vi "Get Column Widths.vi"(8 "error in (no error)":errorcluster, 10 "NewBnds":T1, 11 "Multicolumn List Box View Model In":refnum<class "Process Tree View Model.lvclass">) -> (0 "error out":errorcluster, 2 "Widths":i32[](array[numeric]), 3 "Multicolumn List Box View Model Out":refnum<class "Process Tree View Model.lvclass">)   [LabVIEW 2020, in "Process Tree View Model.lvclass"]
uses:
  Process Tree View Model.lvclass
  <vilib>/Utility/miscctls.llb/LVRectTypeDef.ctl
  Process Tree View Model.lvclass/Process Tree View Model.ctl
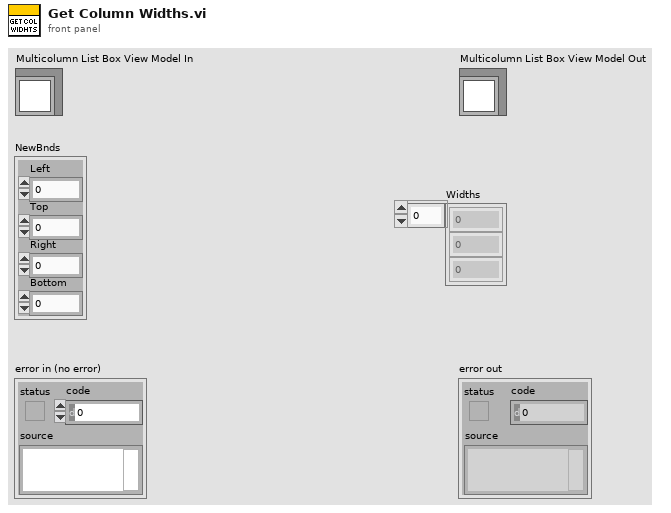
[diagram p1: front panel]
types:
  T1 = typedef "LVRectTypeDef.ctl" = cluster{"Left":i16, "Top":i16, "Right":i16, "Bottom":i16}
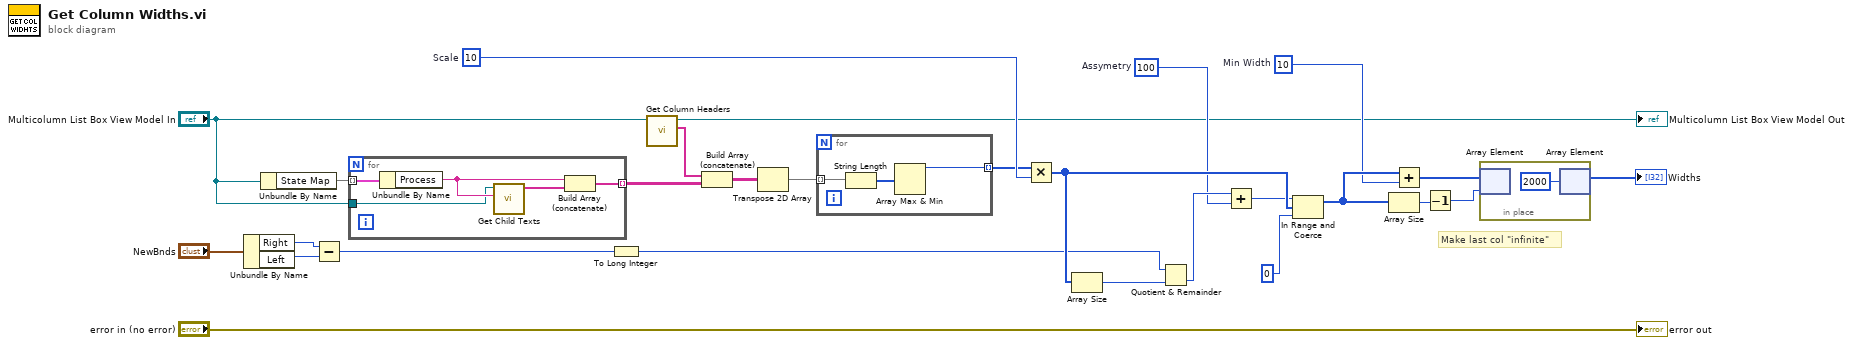
[diagram p0: block diagram]
diagram:
  w9 = 100  # Assymetry
  w11 = 10  # Min Width
  w26 = 10  # Scale
  # "Make last col \"infinite\""
  n1 = Unbundle By Name("NewBnds") -> ("Right"=w20:i16, "Left"=w19:i16)
  n2 = Unbundle By Name("Multicolumn List Box View Model In") -> ("State Map"=w1:map{string, string})
  n3 = Subtract(x=w20, y=w19) -> (x-y=w18:i16)
  n4 = for {
    tunnel: w1 -> [w32] mode=indexing
    tunnel: [w31] -> w7 mode=indexing
    tunnel: "Multicolumn List Box View Model In" -> [w28]
    n5 = Unbundle By Name(w32) -> ("Process"=w30:string)
    n6 = call "Get Child Texts.vi"("Item"=w30, "Process Tree View Model in"=w28) -> ("Texts"=w29:string[])  [unwired: 9 in]
    n7 = Build Array (concatenate)(w30, w29) -> (w31:string[])
  }
  n8 = To Long Integer(number=w18) -> (32bit integer=w16:i32)
  n9 = call "Get Column Headers.vi"("List Box View Model in"="Multicolumn List Box View Model In") -> ("Column Headers"=w2:string[], "List Box View Model out"=→"Multicolumn List Box View Model Out":refnum<class "Process Tree View Model.lvclass">)  [unwired: 8 in, 1 out]
  n10 = Build Array (concatenate)(w2, w7) -> (w5:string[][])
  n11 = Transpose 2D Array(2D array=w5) -> (transposed array=w8:string[][])
  n12 = for {
    tunnel: w8 -> [w35] mode=indexing
    tunnel: [w33] -> w6 mode=indexing
    n13 = String Length(string=w35) -> (length=w34:i32[])
    n14 = Array Max & Min(array=w34) -> (max value=w33:i32)  [unwired: 3 out]
  }
  n15 = Multiply(x=w6, y=w26) -> (x*y=w24:i32[])
  n16 = Array Size(array=w24) -> (size(s)=w13:i32)
  n17 = Quotient & Remainder(x=w16, y=w13) -> (floor(x/y)=w17:i32)  [unwired: 1 out]
  n18 = Add(x=w17, y=w9) -> (x+y=w10:i32)
  n19 = In Range and Coerce(upper limit=w10, x=w24, lower limit=0 ("floor(x/y)")) -> (coerced(x)=w14:i32[])  [unwired: 1 out]
  n20 = Array Size(array=w14) -> (size(s)=w25:i32)
  n21 = Add(x=w14, y=w11) -> (x+y=w12:i32[])
  n22 = Decrement(x=w25) -> (x-1=w22:i32)
  n23 = in-place {
    n24 = in-place-array #1(w12, w22) -> ()  [unwired: 1 out]
    n25 = in-place-array #1(2000 ("element")) -> (→"Widths":i32[])  [unwired: 1 out]
  }
  "error out" <- "error in (no error)"
